vi "Untitled 8.vi"   [LabVIEW 2016]
uses:
  <vilib>/NXT/Block Support/NXT_OutputPort.ctl
  <vilib>/NXT/NXTIO Xnodes/NXTIONodeSubVIs/NXTMoveMotors.vi
  <vilib>/NXT/Dual Mode Library/Waits/Wait_Num.vi
  <vilib>/NXT/Subs/LVHSConnector.ctl
  <vilib>/NXT/NXTIO Xnodes/AddressXNode/NXTIOAddress.xnode
  Documents/LabVIEW Data/NXTRobotics/Projects/Team072DesignChallenge/Team072DesignChallenge.lvrbt
  <vilib>/NXT/NXTIO Xnodes/NXTIOXNode/NXTIO.xnode
  <vilib>/NXT/LegoClasses/BrickReference/BrickReference.lvclass
types:
  T1 = typedef "NXT_OutputPort.ctl" = u8
  T2 = typedef "LVHSConnector.ctl" = refnum<class "BrickReference.lvclass">
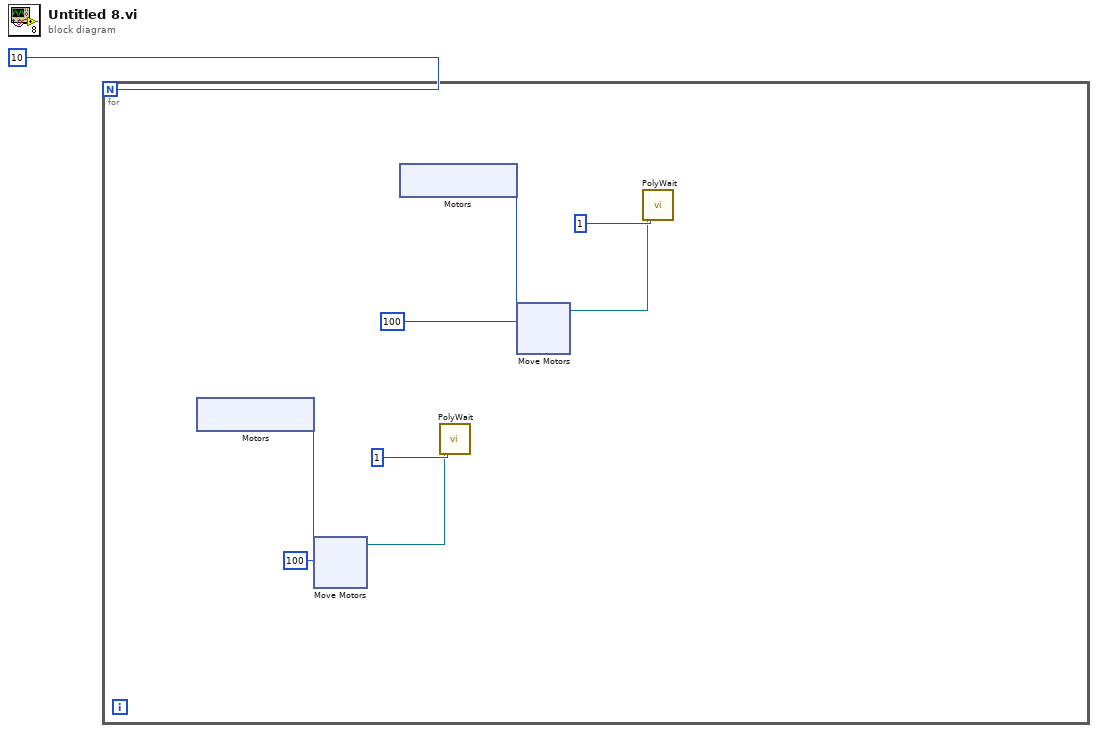
[diagram p0: block diagram]
diagram:
  n1 = for {
    N: 10 -> [_]
    n2 = xnode "Motors"() -> ("Motor"=w9:T1)
    n3 = xnode "Move Motors"("Power/Speed 1"=i8 100, "Motors"=w9) -> ("NXT/EV3"=w7:T2)  [unwired: 1 in]
    n4 = xnode "Motors"() -> ("Motor"=w5:T1)
    n5 = call-poly <vilib>:"PolyWait.vi"("Time (1 sec)"=1, "NXT/EV3"=w7) -> ()  [unwired: 2 in, 1 out]
    n6 = xnode "Move Motors"("Power/Speed 1"=100, "Motors"=w5) -> ("NXT/EV3"=w3:T2)  [unwired: 1 in]
    n7 = call-poly <vilib>:"PolyWait.vi"("Time (1 sec)"=1, "NXT/EV3"=w3) -> ()  [unwired: 2 in, 1 out]
  }
